vi "Do.vi"(8 "error in (no error)":errorcluster, 10 "Actor in":refnum<class "Actor.lvclass">, 11 "Unregister AEs Msg":refnum<class "Unregister AEs Msg.lvclass">) -> (0 "error out":errorcluster, 2 "Actor out":refnum<class "Actor.lvclass">)   [LabVIEW 2015, in "CS++PVMonitor.lvlib" / "Unregister AEs Msg.lvclass"]
doc: "This VI delivers the message to the actor by calling the appropriate method(s) on the actor."
uses:
  Unregister AEs Msg.lvclass
  <vilib>/ActorFramework/Actor/Actor.lvclass
  CS++PVMonitor/CS++PVMonitor.lvclass
  Unregister AEs Msg.lvclass/Unregister AEs Msg.ctl
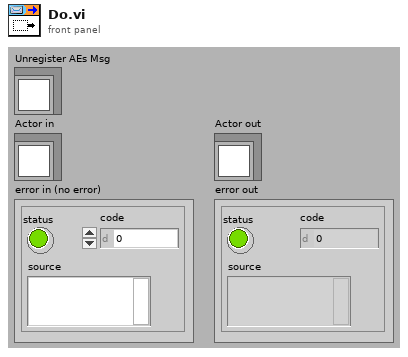
[diagram p1: front panel]
types:
  T1 = cluster{"Self-Enqueuer":refnum<class "Message Enqueuer.lvclass">, "AE URls":string[]}
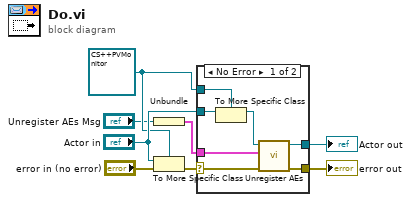
[diagram p0: block diagram]
diagram:
  w3 = refnum<class "CS++PVMonitor.lvclass"> refnum ("Actor in")
  n1 = Unbundle ("Main-Unbundle")("Unregister AEs Msg") -> (w1:T1)
  n2 = To More Specific Class(target class=w3, reference="Actor in", error in="error in (no error)") -> (error out=w7:errorcluster)  [unwired: 1 out]
  n3 = case shown="No Error" w7 {
    selector: w7 -> [w13 w17]
    tunnel: [w15 w17] -> w6
    tunnel: [w14 w16] -> w5
    tunnel: "Actor in" -> [w12 w16]
    tunnel: w3 -> [w11 _]
    tunnel: w1 -> [w9 _]
    frame No Error {
      n4 = To More Specific Class(target class=w11, reference=w12) -> (specific class reference=w10:refnum<class "CS++PVMonitor.lvclass">)  [unwired: 1 in, 1 out]
      n5 = call "Unregister AEs.vi"("error in (no error)"=w13, "Unregister Info"=w9, "CS++PVMonitor in"=w10) -> ("error out"=w15:errorcluster, "CS++PVMonitor out"=w14:refnum<class "CS++PVMonitor.lvclass">)  [unwired: 7 in]
    }
    frame Error {
    }
  }
  "error out" <- w6
  "Actor out" <- w5
